vi "LoopClock.vi"(7 "Instance":i32, 10 "timeout in ms (-1)":i32=-1, 11 "Notifier in":refnum<notifier>) -> ()   [LabVIEW 2017, in "Communication.lvlib"]
uses:
  Communication.lvlib
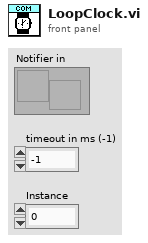
[diagram p1: front panel]
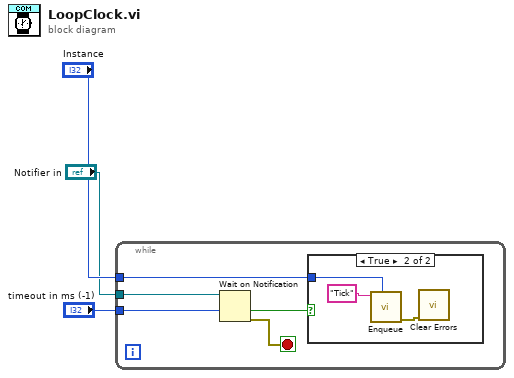
[diagram p0: block diagram]
diagram:
  n1 = while {
    tunnel: "Notifier in" -> [w8]
    tunnel: "timeout in ms (-1)" -> [w6]
    tunnel: "Instance" -> [w4]
    stop <- w7 stop-if-true
    n2 = Wait on Notification(notifier=w8, timeout in ms (-1)=w6) -> (timed out?=w5:bool, error out=w7:errorcluster)  [unwired: 2 in, 2 out]
    n3 = case shown="True" w5 {
      tunnel: w4 -> [_ w10]
      frame False {
      }
      frame True {
        n4 = call "Enqueue.vi"("Instance"=w10, "Msg"="Tick") -> ("error out"=w9:errorcluster)  [unwired: 9 in]
        n5 = call <vilib>:"Clear Errors.vi"("error in (no error)"=w9) -> ()  [unwired: 5 in, 2 out]
      }
    }
  }
